vi "HeaderAction.vi"(0 "InstrClass":refnum<class "ThorPM100A.lvclass"> caption="DNL_LabVIEW Object in", 11 "error in (no error)":errorcluster caption="entrée d'erreur (pas d'erreur)") -> (4 "InstrClassOut":refnum<class "ThorPM100A.lvclass"> caption="DNL_LabVIEW Object out", 6 "DataNames":string[](array[string]), 8 "Instr Name":string, 10 "HeaderString":string, 13 "ArrDisplayNames":string[](array[string]), 14 "DisplayNames":string[](array[string]), 15 "error out":errorcluster caption="sortie d'erreur")   [LabVIEW 2019, in "ThorPM100A.lvclass"]
uses:
  ThorPM100A.lvclass
  C:/Programmes Labview/LabscanV1A/DevicesClass/BaseDevice/BaseDevice.lvclass
  ThorPM100A.lvclass/ThorPM100A.ctl
  BaseDevice/BaseDevice.lvclass
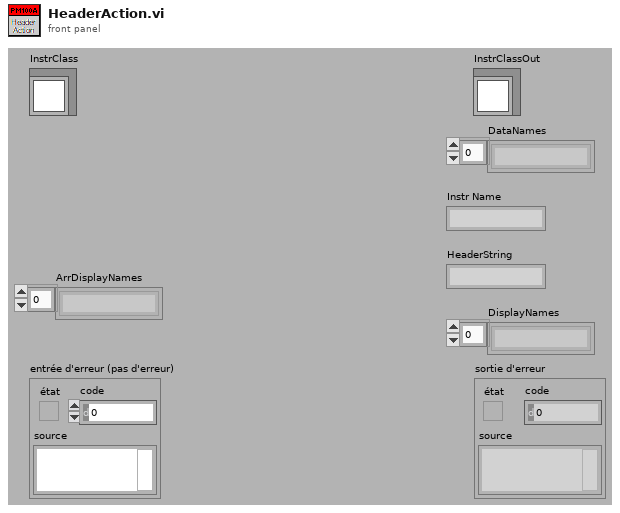
[diagram p1: front panel]
types:
  T1 = typedef "ThorPM100A.lvclass/ThorPM100A_Func.ctl" = enum16{"Read Power (mW)"}
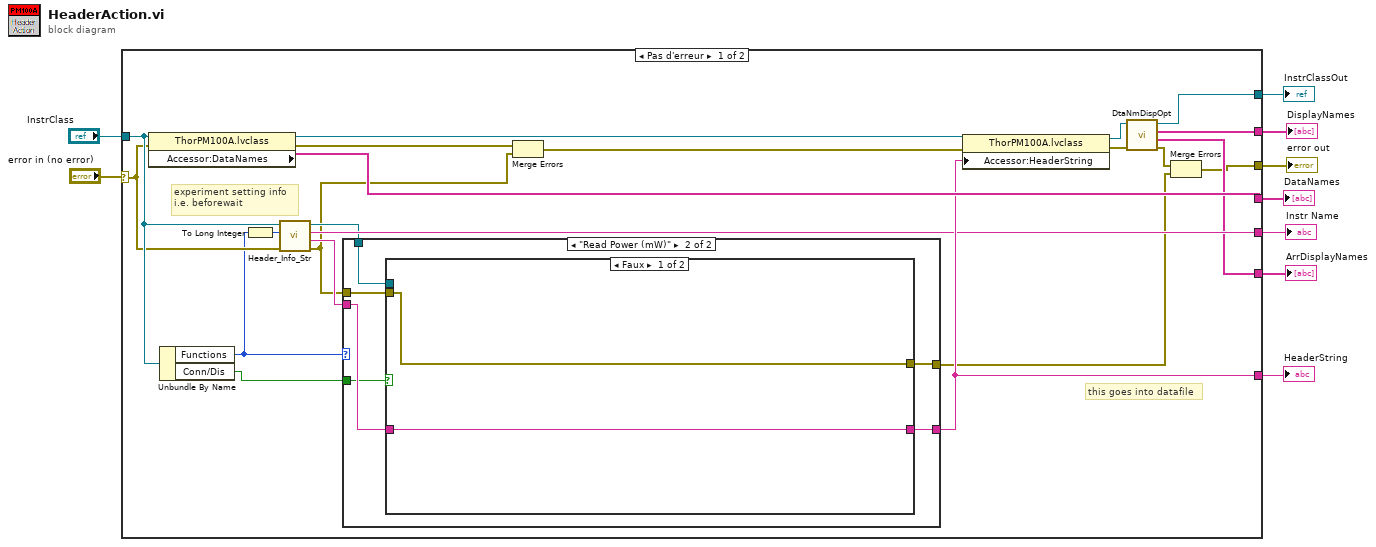
[diagram p0: block diagram]
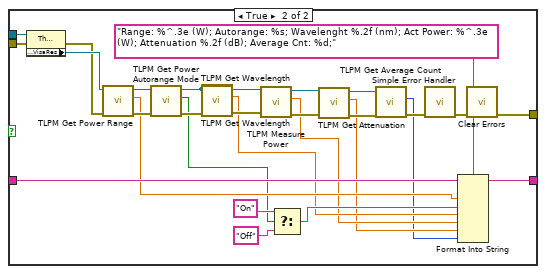
[diagram p3: hidden frame]
diagram:
  n1 = case shown="Pas d'erreur" "error in (no error)" {
    selector: "error in (no error)" -> [w19 w71]
    tunnel: [w28 _] -> w8
    tunnel: [w31 _] -> w7
    tunnel: "InstrClass" -> [w22 w72]
    tunnel: [w12 w71] -> w5
    tunnel: [w25 w72] -> w3
    tunnel: [w21 _] -> w4
    tunnel: [w23 _] -> w2
    tunnel: [w15 _] -> w1
    frame No Error {
      # "this goes into datafile"
      # "experiment setting info\ni.e. beforewait"
      n2 = property class="ThorPM100A.lvclass"(reference=w22, error in=w19) -> (reference out=w30:refnum<class "ThorPM100A.lvclass">, error out=w29:errorcluster, "Accessor:DataNames"=w31:string[])
      n3 = Unbundle By Name(w22) -> ("Functions"=w17:T1, "Conn/Dis"=w10:bool)
      n4 = To Long Integer(number=w17) -> (32bit integer=w16:i32)
      n5 = call-dynamic "Header_Info_Str.vi"("error in (no error)"=w19, "Functions"=w16, "DefaultDev in"=w22) -> ("error out"=w13:errorcluster, "HdrInfoStr"=w20:string, "InstrumentName"=w21:string, "DefaultDev out"=w14:refnum<class "ThorPM100A.lvclass">)  [unwired: 5 in]
      n6 = case shown="\"Read Power (mW)\"" w17 {
        tunnel: [w33 w36] -> w28
        tunnel: w20 -> [w33 w37]
        tunnel: w14 -> [_ w39]
        tunnel: w13 -> [w32 w38]
        tunnel: [w32 w35] -> w11
        tunnel: w10 -> [_ w34]
        frame Default {
        }
        frame "Read Power (mW)" {
          n7 = case shown="Faux" w34 {
            tunnel: w39 -> [_ w66]
            tunnel: w38 -> [w41 w65]
            tunnel: w37 -> [w40 w57]
            tunnel: [w40 w54] -> w36
            tunnel: [w41 w42] -> w35
            frame False {
            }
            frame True {
              n8 = property class="ThorPM100A.lvclass"(reference=w66, error in=w65) -> (error out=w63:errorcluster, "Accessor:VisaRes"=w64:refnum<visa-resource-name>)  [unwired: 1 out]
              n9 = call <instrlib>:"TLPM Get Power Range.vi"("error in (no error)"=w63, "instrument handle"=w64) -> ("error out"=w62:errorcluster, "Power Value"=w52:dbl, "instrument handle out"=w70:refnum<visa-resource-name>)  [unwired: 7 in]
              n10 = call <instrlib>:"TLPM Get Power Autorange Mode.vi"("error in (no error)"=w62, "instrument handle"=w70) -> ("error out"=w61:errorcluster, "Power Autorange Mode"=w49:bool, "instrument handle out"=w67:refnum<visa-resource-name>)  [unwired: 7 in]
              n11 = call <instrlib>:"TLPM Get Wavelength.vi"("error in (no error)"=w61, "instrument handle"=w67) -> ("error out"=w60:errorcluster, "Wavelength"=w47:dbl)  [unwired: 7 in, 1 out]
              n12 = call <instrlib>:"TLPM Get Wavelength.vi"("instrument handle"=w67) -> ("instrument handle out"=w69:refnum<visa-resource-name>)  [unwired: 8 in, 2 out]
              n13 = call <instrlib>:"TLPM Measure Power.vi"("error in (no error)"=w60, "instrument handle"=w69) -> ("error out"=w59:errorcluster, "Power"=w46:dbl, "instrument handle out"=w68:refnum<visa-resource-name>)  [unwired: 7 in]
              n14 = Select(t="On", s=w49, f="Off") -> (s? t:f=w48:string)
              n15 = call <instrlib>:"TLPM Get Attenuation.vi"("error in (no error)"=w59, "instrument handle"=w68) -> ("error out"=w56:errorcluster, "Attenuation"=w45:dbl, "instrument handle out"=w53:refnum<visa-resource-name>)  [unwired: 7 in]
              n16 = call <instrlib>:"TLPM Get Average Count.vi"("error in (no error)"=w56, "instrument handle"=w53) -> ("error out"=w55:errorcluster, "Average Count"=w44:i16)  [unwired: 7 in, 1 out]
              n17 = call <vilib>:"Simple Error Handler.vi"("error in (no error)"=w55) -> ("error out"=w43:errorcluster)  [unwired: 4 in, 4 out]
              n18 = Format Into String(format string="Range: %^.3e (W); Autorange: %s; Wavelenght %.2f (nm); Act Power: %^.3e (W); Attenuation %.2f (dB); Average Cnt: %d;" ("chaîne de format"), initial string=w57, w52, w48, w47, w46, w45, w44) -> (resulting string=w54:string)  [unwired: 1 in, 1 out]
              n19 = call <vilib>:"Clear Errors.vi"("error in (no error)"=w43) -> ("error out"=w42:errorcluster)  [unwired: 5 in, 1 out]
            }
          }
        }
      }
      n20 = Merge Errors(w29, w13) -> (w18:errorcluster)
      n21 = property class="ThorPM100A.lvclass"(reference=w30, error in=w18, "Accessor:HeaderString"=w28) -> (reference out=w24:refnum<class "ThorPM100A.lvclass">, error out=w27:errorcluster)
      n22 = call "DtaNmDispOpt.vi"("error in (no error)"=w27, "BaseDevice en entrée"=w24) -> ("error out"=w26:errorcluster, "ArrDisplayNames"=w15:string[], "DisplayNames"=w23:string[], "BaseDevice en sortie"=w25:refnum<class "ThorPM100A.lvclass">)  [unwired: 6 in]
      n23 = Merge Errors(w26, w11) -> (w12:errorcluster)
    }
    frame Error {
    }
  }
  "error out" <- w5
  "InstrClassOut" <- w3
  "DataNames" <- w7
  "HeaderString" <- w8
  "Instr Name" <- w4
  "DisplayNames" <- w2
  "ArrDisplayNames" <- w1
